vi "MakeWave.vi"(0 "Instrument Resource Name":refnum<visa-resource-name>="GPIB::10::INSTR", 1 "exp per cycle  (ms) sg":sgl=0.2 format="%.3f", 2 "PRF (Hz) sg":dbl=1000.0 caption="PRF (Hz)", 3 "error in (no error)":errorcluster, 4 "2nd Busrt Scale":dbl=0.5) -> (5 "Custom wave":waveform(i16)(graph), 6 "output waveform":waveform(i16))   [LabVIEW 2022 SP3]
uses:
  <vilib>/measure/NI_MABase.lvlib
panel:
  in  "Case Constant\n(See Context Help)":bool=TRUE
  out "Free Memory Slots":i32
  in  "User Def. Wfm Name":string="JEFFWAVE"
  out "error out":errorcluster
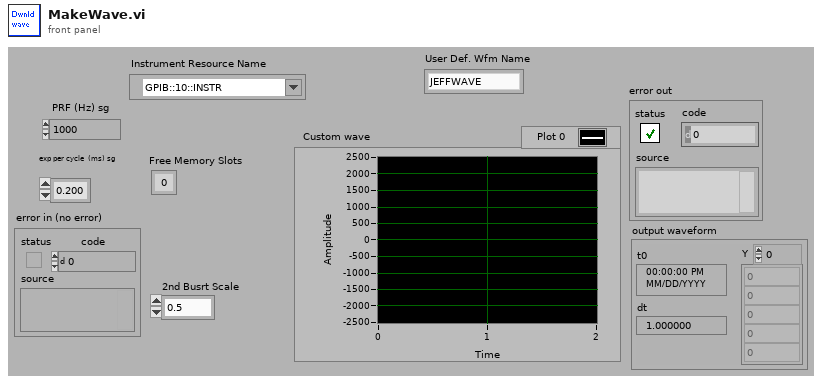
[diagram p1: front panel]
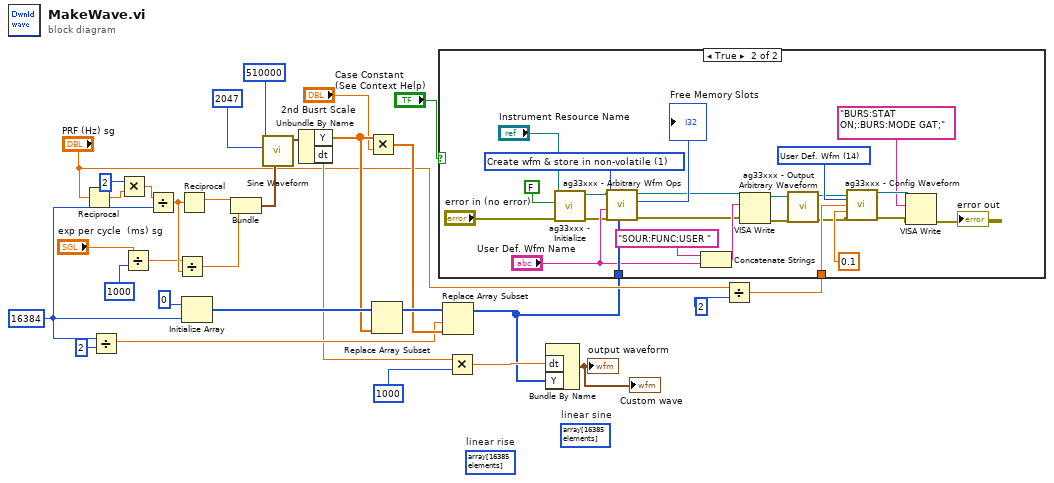
[diagram p0: block diagram]
diagram:
  (unwired) i16[] array[16385 elements]  # linear rise
  (unwired) i16[] array[16385 elements]  # linear sine
  w19 = i16 16384
  n1 = Reciprocal(x="PRF (Hz) sg") -> (1/x=w7:dbl)
  n2 = Divide(x=w19, y=2) -> (x/y=w18:dbl)
  n3 = Multiply(x=2, y=w7) -> (x*y=w5:dbl)
  n4 = Divide(x="exp per cycle  (ms) sg", y=1000) -> (x/y=w16:sgl)
  n5 = Divide(x=w5, y=w19) -> (x/y=w29:dbl)
  n6 = Divide(x=w16, y=w29) -> (x/y=w14:dbl)
  n7 = Reciprocal(x=w29) -> (1/x=w27:dbl)
  n8 = Initialize Array(i16 0, w19) -> (w23:i16[])
  n9 = Bundle(w27, w14) -> (w28:cluster{dbl, dbl})  [unwired: 1 out]
  n10 = call <vilib>:"Sine Waveform.vi"("sampling info"=w28, "amplitude"=2047, "frequency"=510000) -> ("signal out"=w24:waveform(dbl))  [unwired: 4 in, 4 out]
  n11 = Unbundle By Name(w24) -> ("Y"=w22:dbl[], "dt"=w12:dbl)
  n12 = Multiply(x=w22, y="2nd Busrt Scale") -> (x*y=w20:dbl[])
  n13 = Replace Array Subset(array=w23, new element=w22) -> (w21:i16[])  [unwired: 1 in]
  n14 = Replace Array Subset(array=w21, new element=w20, index=w18) -> (w1:i16[])
  n15 = Multiply(x=w12, y=1000) -> (x*y=w11:dbl)
  n16 = Bundle By Name("dt"=w11, "Y"=w1) -> (→"Custom wave" →"output waveform":waveform(i16))  [unwired: 1 out]
  n17 = Divide(x="PRF (Hz) sg", y=2) -> (x/y=w3:dbl)
  n18 = case shown="True" "Case Constant\n(See Context Help)" {
    tunnel: w3 -> [_ w52]
    tunnel: w1 -> [_ w50]
    frame False {
    }
    frame True {
      w53 = u16 14 items=["DC"=0, "Sine"=1, "Square"=2, "Triangle"=3, "Ramp"=4, "Pulse"=6, "Noise"=7, "Sinc"=8, "Neg. Ramp"=9, "Exp. Rise"=10, "Exp. Fall"=11, "Cardiac"=12, "Volatile"=13, "User Def. Wfm"=14] ("Waveform Shape (1: Sine)")
      w55 = u16 1 items=["Create wfm & store in volatile", "Create wfm & store in non-volatile", "Copy wfm from volatile", "Delete wfm from volatile", "Delete one wfm from non-volatile", "Delete all wfms from non-volatile"] ("Mode (0: Create wfm & store in volatile)")
      n19 = call <instrlib>:"ag33xxx - Initialize.vi"("error in (no error)"="error in (no error)", "ID Query (T: Check)"=FALSE, "Instrument Resource Name"="Instrument Resource Name") -> ("error out"=w42:errorcluster, "dup VISA session"=w43:refnum<visa-resource-name>)  [unwired: 1 in, 6 out]
      n20 = call <instrlib>:"ag33xxx - Arbitrary Wfm Ops.vi"("Data"=w50, "error in (no error)"=w42, "Waveform Name"="User Def. Wfm Name", "Mode (0: Create wfm & store in volatile)"=w55, "VISA session"=w43) -> ("error out"=w40:errorcluster, "Free Memory Slots"=→"Free Memory Slots":i32, "dup VISA session"=w41:refnum<visa-resource-name>)  [unwired: 4 out]
      n21 = Concatenate Strings("SOUR:FUNC:USER ", "User Def. Wfm Name") -> (w44:string)
      n22 = VISA Write(VISA resource name=w41, write buffer=w44, error in (no error)=w40) -> (VISA resource name out=w39:refnum<visa-resource-name>, error out=w38:errorcluster)  [unwired: 1 out]
      n23 = call <instrlib>:"ag33xxx - Output Arbitrary Waveform.vi"("error in (no error)"=w38, "VISA session"=w39) -> ("error out"=w47:errorcluster, "dup VISA session"=w48:refnum<visa-resource-name>)  [unwired: 8 out]
      n24 = call <instrlib>:"ag33xxx - Config Waveform.vi"("VISA session"=w48, "Waveform Shape (1: Sine)"=w53, "Frequency (1000 Hz)"=w52, "Amplitude (0.1 Vpp)"=0.1, "error in (no error)"=w47) -> ("dup VISA session"=w37:refnum<visa-resource-name>, "error out"=w36:errorcluster)  [unwired: 2 in, 7 out]
      n25 = VISA Write(VISA resource name=w37, write buffer="BURS:STAT ON;:BURS:MODE GAT;", error in (no error)=w36) -> (error out=→"error out":errorcluster)  [unwired: 2 out]
    }
  }
